vi "constructor.vi"(1 "element_num":u32, 2 "initial_element":dbl format="%#_13g") -> (0 "output_double_array.lvclass":refnum<class "double_array.lvclass">)   [LabVIEW 2014, in "double_array.lvclass"]
uses:
  double_array.lvclass
  double_array.lvclass/double_array.ctl
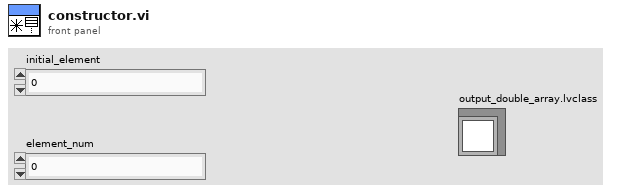
[diagram p1: front panel]
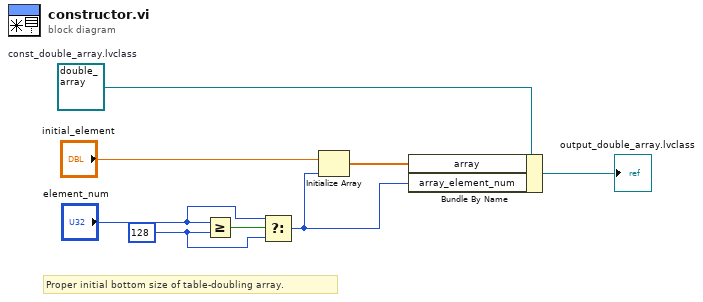
[diagram p0: block diagram]
diagram:
  w4 = refnum<class "double_array.lvclass"> refnum  # const_double_array.lvclass
  w6 = u32 128 ("y")
  # "Proper initial bottom size of table-doubling array."
  n1 = Greater Or Equal?(x="element_num", y=w6) -> (x >= y?=w8:bool)
  n2 = Select(t="element_num", s=w8, f=w6) -> (s? t:f=w2:u32)
  n3 = Initialize Array("initial_element", w2) -> (w3:dbl[])
  n4 = Bundle By Name(cluster=w4, "array"=w3, "array_element_num"=w2) -> (→"output_double_array.lvclass":refnum<class "double_array.lvclass">)
